vi "medicaoTemperatura.vi"() -> (3 "data":dbl)   [LabVIEW 2012]
panel:
  out "Waveform Chart":dynamicdata(graph)
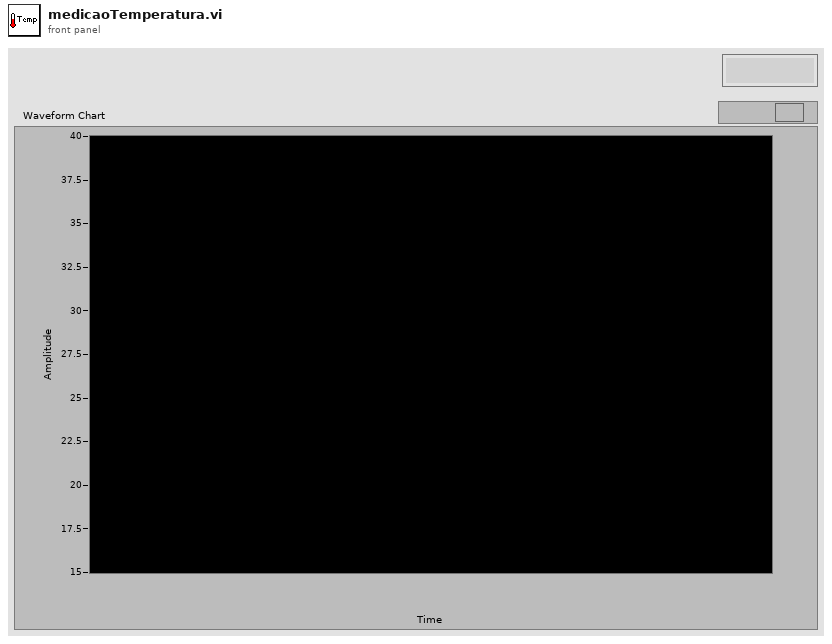
[diagram p1: front panel]
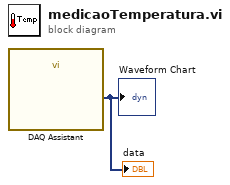
[diagram p0: block diagram]
diagram:
  n1 = call "DAQ Assistant"() -> ("data"=→"Waveform Chart" →"data":dynamicdata)  [unwired: 17 in, 2 out]
